vi "Limelight Set Pipeline Number.vi"(11 "Pipeline Number":i8=1 min=0 max=9 step=1) -> (0 "error out":errorcluster)   [LabVIEW 2019]
uses:
  <vilib>/Rock Robotics/Network Tables/NT Write Number.vi
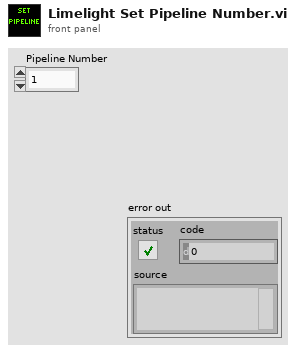
[diagram p1: front panel]
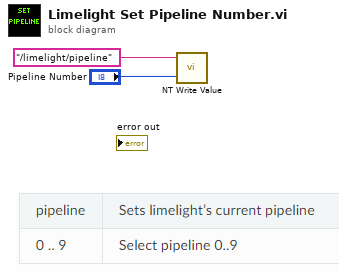
[diagram p0: block diagram]
diagram:
  n1 = call-poly <vilib>:"NT Write Value.vi"("Numeric"="Pipeline Number", "Name"="/limelight/pipeline") -> ()  [unwired: 9 in, 1 out]
